vi "Save Image.vi"(8 "Data":dbl[][](array[numeric]), 9 "Na/Rb (0/1)":u8, 10 "Process Index":u8, 11 "Current File Num":u16) -> ()   [LabVIEW 2015]
panel:
  out "Path":path
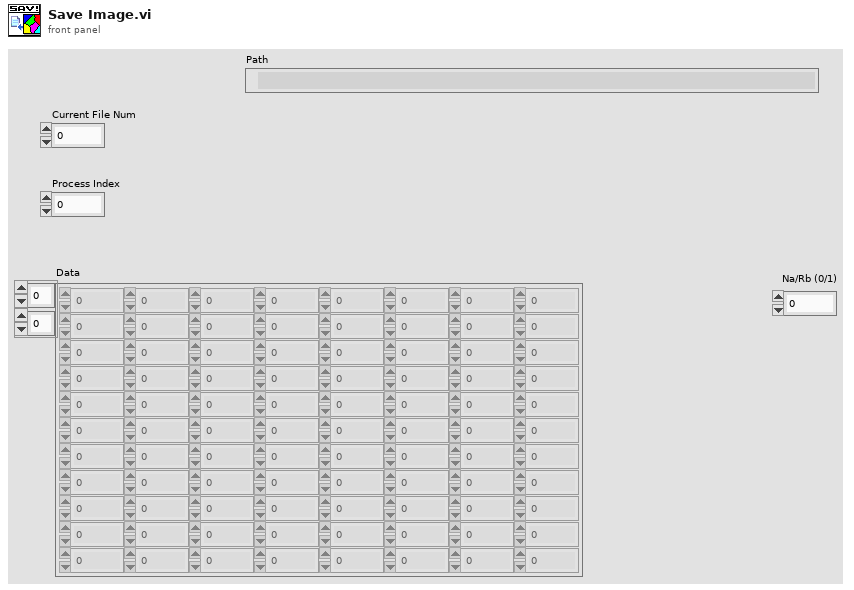
[diagram p1: front panel]
types:
  T1 = typedef "Image Type" = u32
  T2 = typedef "IMAQ Image.ctl" = refnum<image>
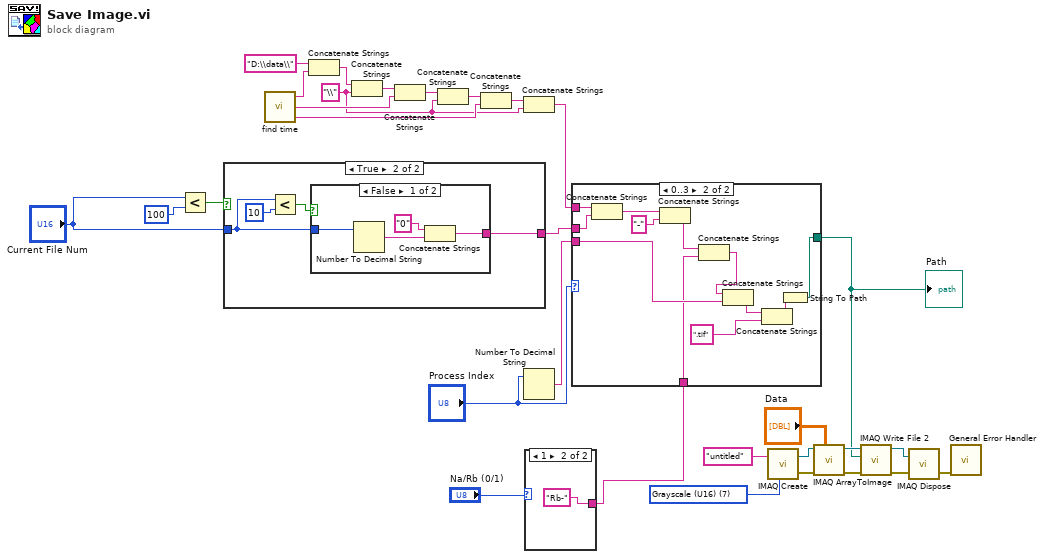
[diagram p0: block diagram]
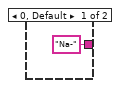
[diagram p2: hidden frame]
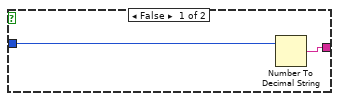
[diagram p3: hidden frame]
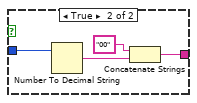
[diagram p4: hidden frame]
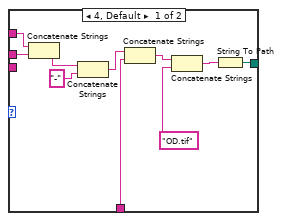
[diagram p5: hidden frame]
diagram:
  w11 = "\\" ("字符串")
  w23 = T1 7 items=["Grayscale (U8)", "Grayscale (I16)", "Grayscale (SGL)", "Complex (CSG)", "RGB (U32)", "HSL (U32)", "RGB (U64)", "Grayscale (U16)"] ("Image Type")
  n1 = Less?(x="Current File Num", y=u16 100) -> (x < y?=w3:bool)
  n2 = case shown="True" w3 {
    tunnel: "Current File Num" -> [w32 w34]
    tunnel: [w31 w33] -> w9
    frame False {
      n3 = Number To Decimal String(number=w32) -> (decimal integer string=w31:string)  [unwired: 1 in]
    }
    frame True {
      n4 = Less?(x=w34, y=u16 10) -> (x < y?=w35:bool)
      n5 = case shown="False" w35 {
        tunnel: w34 -> [w39 w44]
        tunnel: [w37 w41] -> w33
        frame False {
          n6 = Number To Decimal String(number=w39) -> (decimal integer string=w38:string)  [unwired: 1 in]
          n7 = Concatenate Strings("0" ("字符串"), w38) -> (w37:string)
        }
        frame True {
          n8 = Number To Decimal String(number=w44) -> (decimal integer string=w42:string)  [unwired: 1 in]
          n9 = Concatenate Strings("00" ("字符串"), w42) -> (w41:string)
        }
      }
    }
  }
  n10 = call "find time.vi"() -> ("day"=w13:string, "month"=w16:string, "year"=w19:string)  [unwired: 3 in]
  n11 = Concatenate Strings("D:\\data\\", w19) -> (w18:string)
  n12 = Concatenate Strings(w18, w11) -> (w17:string)
  n13 = Concatenate Strings(w17, w16) -> (w15:string)
  n14 = Concatenate Strings(w15, w11) -> (w14:string)
  n15 = Concatenate Strings(w14, w13) -> (w12:string)
  n16 = Concatenate Strings(w12, w11) -> (w8:string)
  n17 = Number To Decimal String(number="Process Index") -> (decimal integer string=w10:string)  [unwired: 1 in]
  n18 = case shown="1" "Na/Rb (0/1)" {
    tunnel: ["Na-" ("字符串") "Rb-" ("字符串")] -> w1
    frame 0, Default {
    }
    frame 1 {
    }
  }
  n19 = case shown="0..3" "Process Index" {
    tunnel: [w51 w68] -> w7
    tunnel: w9 -> [w54 w67]
    tunnel: w10 -> [_ w64]
    tunnel: w8 -> [w50 w63]
    tunnel: w1 -> [w47 w58]
    frame 4, Default {
      n20 = Concatenate Strings(w50, w54) -> (w56:string)
      n21 = Concatenate Strings(w56, "-" ("字符串")) -> (w49:string)
      n22 = Concatenate Strings(w49, w47) -> (w48:string)
      n23 = Concatenate Strings(w48, "OD.tif" ("字符串")) -> (w52:string)
      n24 = String To Path(string=w52) -> (path=w51:path)
    }
    frame 0..3 {
      n25 = Concatenate Strings(w63, w67) -> (w66:string)
      n26 = Concatenate Strings(w66, "-" ("字符串")) -> (w59:string)
      n27 = Concatenate Strings(w59, w58) -> (w57:string)
      n28 = Concatenate Strings(w57, w64) -> (w62:string)
      n29 = Concatenate Strings(w62, ".tif" ("字符串")) -> (w60:string)
      n30 = String To Path(string=w60) -> (path=w68:path)
    }
  }
  "Path" <- w7
  n31 = call "IMAQ Create"("Image Name"="untitled", "Image Type"=w23) -> ("New Image"=w21:T2, "error out"=w22:errorcluster)  [unwired: 3 in]
  n32 = call "IMAQ ArrayToImage"("Image Pixels (U16)"="Data", "error in (no error)"=w22, "Image"=w21) -> ("error out"=w26:errorcluster, "Image Out"=w29:T2)  [unwired: 7 in]
  n33 = call-poly "IMAQ Write File 2"("error in (no error)"=w26, "File Path"=w7, "Image"=w29) -> ("error out"=w27:errorcluster, "Image Out (duplicate)"=w28:T2)  [unwired: 7 in]
  n34 = call "IMAQ Dispose"("Image"=w28, "error in (no error)"=w27) -> ("error out"=w24:errorcluster)  [unwired: 4 in]
  n35 = call <vilib>:"General Error Handler.vi"("error in (no error)"=w24) -> ()  [unwired: 10 in, 5 out]
